vi "gRPC to LV Timestamp.vi"(11 "gRPC Timestamp":T1) -> (3 "LV Timestamp":timestamp)   [LabVIEW 2023, in "gRPC Client.lvclass"]
uses:
  gRPC Client.lvclass
  gRPC Client.lvclass/gRPC Client.ctl
  Generated_client/RPC Messages/google_protobuf_Timestamp.ctl
  Generated_client/Generated_client.lvlib
panel:
  # "Connector Pane"
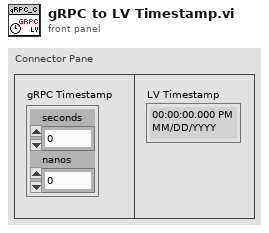
[diagram p1: front panel]
types:
  T1 = typedef "Generated_client.lvlib/google_protobuf_Timestamp.ctl" = cluster{"seconds":i64, "nanos":i32}
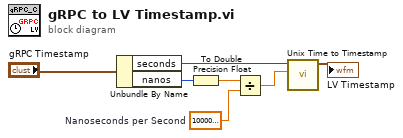
[diagram p0: block diagram]
diagram:
  w6 = 1000000000.0  # Nanoseconds per Second
  n1 = Unbundle By Name("gRPC Timestamp") -> ("seconds"=w3:i64, "nanos"=w4:i32)
  n2 = To Double Precision Float(number=w4) -> (double precision float=w5:dbl)
  n3 = Divide(x=w5, y=w6) -> (x/y=w7:dbl)
  n4 = call <vilib>:"Unix Time to Timestamp.vi"("Fractional Second"=w7, "Unix Time (s)"=w3) -> ("Timestamp"=→"LV Timestamp":timestamp)  [unwired: 8 in, 1 out]
